vi "STTest.vi"(8 "error in":errorcluster caption="错误输入", 9 "React":string="create auto test task", 10 "CMDIn":string="testmode(1)", 11 "ComIn":refnum<visa-resource-name>) -> (0 "error out":errorcluster caption="错误输出", 1 "OK?":bool, 2 "ReactStr":string, 3 "ComOut":refnum<visa-resource-name>)   [LabVIEW 2013]
uses:
  Global.vi
  <vilib>/Instr/_visa.llb/VISA Flush IO Buffer Mask.ctl
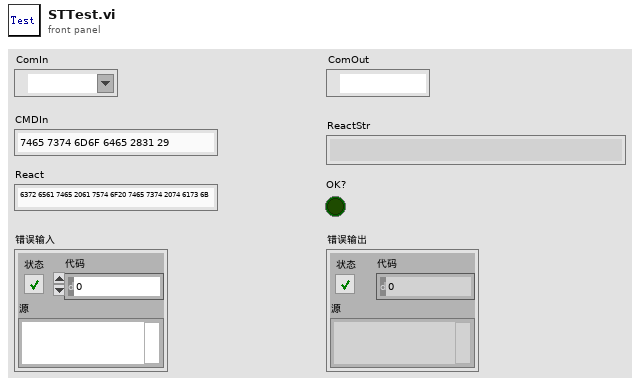
[diagram p1: front panel]
types:
  T1 = typedef "VISA Flush IO Buffer Mask.ctl" = u16
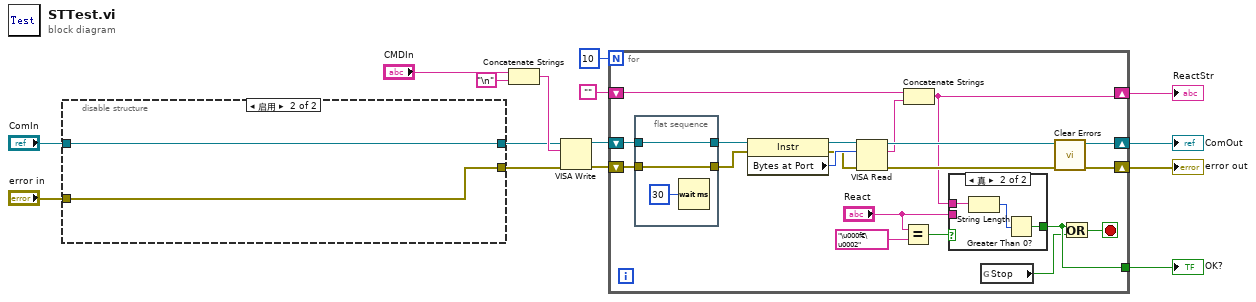
[diagram p0: block diagram]
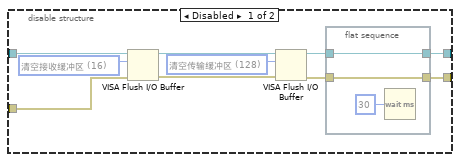
[diagram p2: hidden frame]
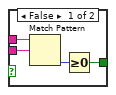
[diagram p3: hidden frame]
diagram:
  n1 = disable-structure shown="启用" {
    disable-tunnel: [w24 w30] -> w7
    disable-tunnel: [w23 w29] -> w6
    disable-tunnel: "ComIn" -> [w21 w30]
    disable-tunnel: "error in" -> [w20 w29]
    frame Disabled {
      w17 = T1 128 items=["清空接收缓冲区"=16, "向设备写入传输缓冲区"=32, "清空接收缓冲区（无I/O）"=64, "清空传输缓冲区"=128] ("Mask")
      w19 = T1 16 items=["清空接收缓冲区"=16, "向设备写入传输缓冲区"=32, "清空接收缓冲区（无I/O）"=64, "清空传输缓冲区"=128] ("Mask")
      n2 = VISA Flush I/O Buffer(VISA resource name=w21, mask (16)=w19, error in (no error)=w20) -> (VISA resource name out=w18:refnum<visa-resource-name>, error out=w16:errorcluster)
      n3 = VISA Flush I/O Buffer(VISA resource name=w18, mask (16)=w17, error in (no error)=w16) -> (VISA resource name out=w25:refnum<visa-resource-name>, error out=w22:errorcluster)
      n4 = flat-sequence {
        tunnel: w25 -> [w28]
        tunnel: [w28] -> w24
        tunnel: [w27] -> w23
        tunnel: w22 -> [w27]
        frame #0 {
          n5 = Wait (ms)(milliseconds to wait=u32 30 ("等待时间（毫秒）")) -> ()  [unwired: 1 out]
        }
      }
    }
    frame Enabled {
    }
  }
  n6 = Concatenate Strings("CMDIn", "\n") -> (w14:string)
  n7 = VISA Write(VISA resource name=w7, write buffer=w14, error in (no error)=w6) -> (VISA resource name out=w12:refnum<visa-resource-name>, error out=w11:errorcluster)  [unwired: 1 out]
  n8 = for {
    N: 10 -> [_]
    shift-right: [w44] -> w3
    shift-left: w12 -> [w49]
    shift-right: [w35] -> w1
    shift-left: w11 -> [w48]
    shift-right: [w40] -> w2
    shift-left: "" -> [w41]
    tunnel: [w39] -> w8
    stop <- w37 stop-if-true
    n9 = flat-sequence {
      tunnel: w49 -> [w59]
      tunnel: w48 -> [w58]
      tunnel: [w59] -> w47
      tunnel: [w58] -> w46
      frame #0 {
        n10 = Wait (ms)(milliseconds to wait=u32 30 ("等待时间（毫秒）")) -> ()  [unwired: 1 out]
      }
    }
    n11 = property class="Instr"(reference=w47, error in=w46) -> (reference out=w45:refnum<visa-resource-name>, error out=w34:errorcluster, "Bytes at Port"=w36:u32)
    n12 = VISA Read(VISA resource name=w45, byte count=w36, error in (no error)=w34) -> (VISA resource name out=w44:refnum<visa-resource-name>, read buffer=w42:string, error out=w43:errorcluster)  [unwired: 1 out]
    n13 = Equal?(x="React", y="\u000f€\u0002" ("React 2")) -> (x = y?=w31:bool)
    n14 = Concatenate Strings(w41, w42) -> (w40:string)
    n15 = case shown="真" w31 {
      tunnel: w40 -> [w53 w56]
      tunnel: [w51 w55] -> w39
      tunnel: "React" -> [w50 _]
      frame False {
        n16 = Match Pattern(string=w53, regular expression=w50) -> (offset past match=w52:i32)  [unwired: 1 in, 3 out]
        n17 = Greater Or Equal To 0?(x=w52) -> (x >= 0?=w51:bool)
      }
      frame True {
        n18 = String Length(string=w56) -> (length=w54:i32)
        n19 = Greater Than 0?(x=w54) -> (x > 0?=w55:bool)
      }
    }
    n20 = global read "Global.vi" "Stop"() -> (w38:bool)
    n21 = call <vilib>:"Clear Errors.vi"("error in (no error)"=w43) -> ("error out"=w35:errorcluster)  [unwired: 6 in]
    n22 = Or(x=w39, y=w38) -> (x .or. y?=w37:bool)
  }
  "error out" <- w1
  "OK?" <- w8
  "ComOut" <- w3
  "ReactStr" <- w2
